vi "VI.GetLibraries.Members.vi"(8 "error in":errorcluster, 10 "All Facade VIs":string[](array[string]), 11 "VI Refnum":refnum<vi>) -> (0 "error out":errorcluster, 1 "Libraries Refnum":refnum<vi>[](array[refnum]), 2 "VI Names":string[](array[string]), 3 "VI Refnum Out":refnum<vi>)   [LabVIEW 2011]
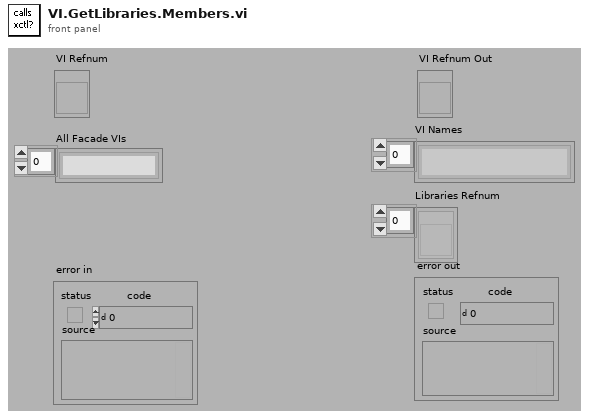
[diagram p1: front panel]
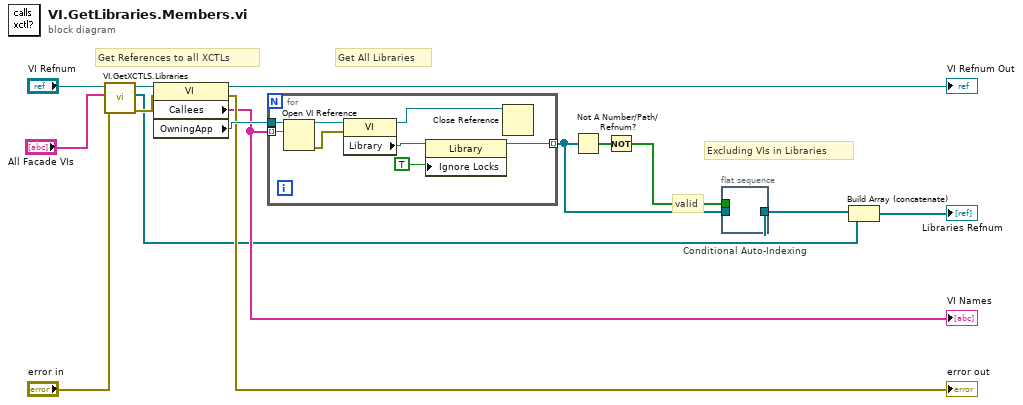
[diagram p0: block diagram]
diagram:
  # "valid"
  # "Excluding VIs in Libraries"
  # "Get All Libraries"
  # "Get References to all XCTLs"
  n1 = call "VI.GetXCTLS.Libraries.vi"("error in"="error in", "All Facade VIs"="All Facade VIs", "vi reference"="VI Refnum") -> ("error out"=w10:errorcluster, "Libraries"=w5:refnum<vi>[], "vi reference out"=w13:refnum<vi>)  [unwired: 6 in]
  n2 = property class="VI"(reference=w13, error in=w10) -> (reference out=→"VI Refnum Out":refnum<vi>, error out=→"error out":errorcluster, "Callees"=w6:string[], "OwningApp"=w11:refnum<vi>)
  "VI Names" <- w6
  n3 = for {
    tunnel: w6 -> [w23] mode=indexing
    tunnel: [w16] -> w4 mode=indexing
    tunnel: w11 -> [w20]
    n4 = Open VI Reference(application reference (local)=w20, vi path=w23) -> (vi reference=w21:refnum<vi>, error out=w22:errorcluster)  [unwired: 4 in]
    n5 = property class="VI"(reference=w21, error in=w22) -> (reference out=w19:refnum<vi>, "Library"=w17:refnum<vi>)  [unwired: 1 out]
    n6 = property class="Library"(reference=w17, "Ignore Locks"=TRUE) -> (reference out=w16:refnum<vi>)  [unwired: 1 in, 1 out]
    n7 = Close Reference(reference=w19) -> ()  [unwired: 1 in, 1 out]
  }
  n8 = Not A Number/Path/Refnum?(number/path/refnum=w4) -> (NaN/Path/Refnum?=w3:bool[])
  n9 = Not(x=w3) -> (.not. x?=w2:bool[])
  n10 = flat-sequence "Conditional Auto-Indexing" {
    tunnel: w2 -> [w26]
    tunnel: w4 -> [w25]
    tunnel: [w24] -> w8
    frame #0 {
      n11 = Boolean To (0,1)(Boolean=w26) -> (0, 1=w29:i16[])
      n12 = To Unsigned Long Integer(number=w29) -> (unsigned 32bit integer=w30:u32[])
      n13 = Add Array Elements(numeric array=w30) -> (sum=w28:u32)
      n14 = for {
        N: w28 -> [_]
        tunnel: w25 -> [w33]
        tunnel: w26 -> [w37]
        shift-right: [w34] -> _
        shift-left: -1 ("start index (0)") -> [w35]
        tunnel: [w32] -> w24 mode=indexing
        # "index out that element"
        # "Find the next element to keep"
        n15 = Increment(x=w35) -> (x+1=w31:i32)
        n16 = Search 1D Array(1D array=w37, element=TRUE, start index (0)=w31) -> (index of element=w34:i32)
        n17 = Index Array(array=w33, index=w34) -> (element=w32:refnum<vi>)
      }
    }
  }
  n18 = Build Array (concatenate)(w8, w5) -> (→"Libraries Refnum":refnum<vi>[])
